vi "MotorGo.vi"(2 "Go!":refnum<k4>, 3 "Motor":string="PI1-SHUTTER", 9 "error in (no error)":errorcluster) -> (0 "Motor out":string="PI1-SHUTTER", 6 "error out":errorcluster)   [LabVIEW 2009]
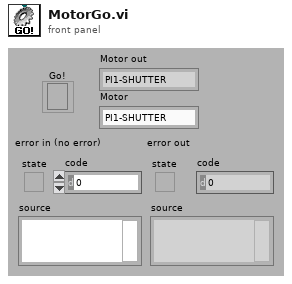
[diagram p1: front panel]
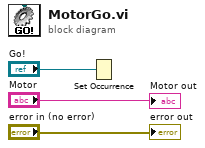
[diagram p0: block diagram]
diagram:
  n1 = Set Occurrence("Go!") -> ()
  "error out" <- "error in (no error)"
  "Motor out" <- "Motor"
